vi "Graph Value to IMAQ Image.vi"(7 "Gray?":bool, 8 "error in":errorcluster, 11 "Intensity Graph Refnum":refnum<vi>) -> (0 "error out":errorcluster, 3 "IMAQ Image":T1)   [LabVIEW 2025, in "Base Graph.lvclass"]
uses:
  Base Graph.lvclass
  <vilib>/vision/Image Controls.llb/IMAQ Image.ctl
  Open-Xml-LabVIEW/Common-Labview-helpers/Source/Common Helpers.lvlib
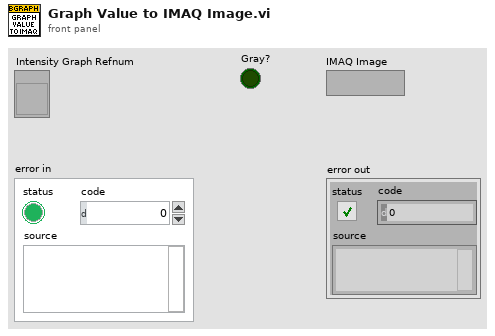
[diagram p1: front panel]
types:
  T1 = typedef "IMAQ Image.ctl" = refnum<image>
  T2 = typedef "Image Type" = u32
  T3 = typedef "imagedata.ctl" = cluster{"image type":i32, "image depth":i32, "image":u8[], "mask":u8[], "colors":u32[], "Rectangle":cluster{"left":i16, "top":i16, "right":i16, "bottom":i16}}
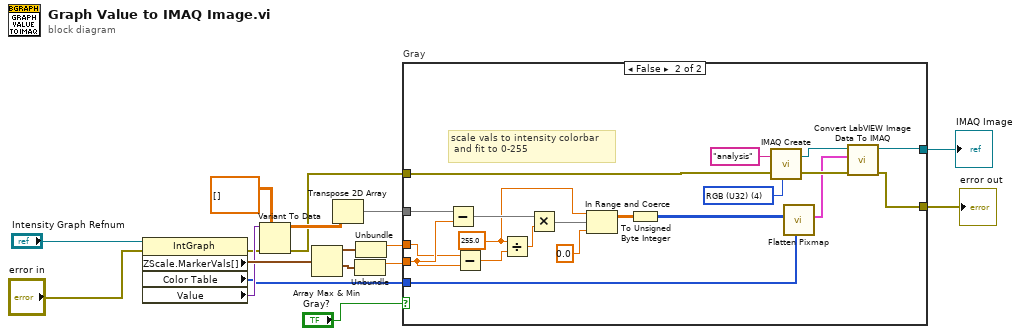
[diagram p0: block diagram]
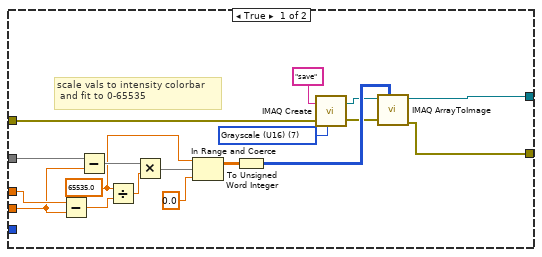
[diagram p2: hidden frame]
diagram:
  n1 = property class="IntGraph"(reference="Intensity Graph Refnum", error in="error in") -> (error out=w11:errorcluster, "ZScale.MarkerVals[]"=w14:cluster{dbl, u32}[], "Color Table"=w2:u32[], "Value"=w12:variant)  [unwired: 1 out]
  n2 = Variant To Data(error in=w11, type=dbl[][] [], Variant=w12) -> (data=w10:dbl[][], error out=w5:errorcluster)
  n3 = Array Max & Min(array=w14) -> (max value=w15:cluster{dbl, u32}, min value=w16:cluster{dbl, u32})  [unwired: 2 out]
  n4 = Transpose 2D Array(2D array=w10) -> (transposed array=w6:dbl[][])
  n5 = Unbundle(w16) -> (w8:dbl)  [unwired: 1 out]
  n6 = Unbundle(w15) -> (w7:dbl)  [unwired: 1 out]
  n7 = case "Gray" shown="False" "Gray?" {
    tunnel: w6 -> [w27 w47]
    tunnel: w5 -> [w26 w46]
    tunnel: [w25 w36] -> w3
    tunnel: [w24 w37] -> w4
    tunnel: w8 -> [w22 w45]
    tunnel: w7 -> [w23 w44]
    tunnel: w2 -> [_ w41]
    frame True {
      w18 = T2 7 items=["Grayscale (U8)", "Grayscale (I16)", "Grayscale (SGL)", "Complex (CSG)", "RGB (U32)", "HSL (U32)", "RGB (U64)", "Grayscale (U16)"] ("Image Type")
      w31 = 65535.0
      # "scale vals to intensity colorbar\n and fit to 0-65535"
      n8 = Subtract(x=w23, y=w22) -> (x-y=w34:dbl)
      n9 = Subtract(x=w27, y=w22) -> (x-y=w35:dbl[][])
      n10 = Divide(x=w31, y=w34) -> (x/y=w33:dbl)
      n11 = Multiply(x=w35, y=w33) -> (x*y=w30:dbl[][])
      n12 = In Range and Coerce(upper limit=w31, x=w30, lower limit=0.0) -> (coerced(x)=w29:dbl[][])  [unwired: 1 out]
      n13 = To Unsigned Word Integer(number=w29) -> (unsigned 16bit integer=w28:u16[][])
      n14 = call "IMAQ Create"("Image Name"="save", "Image Type"=w18, "error in (no error)"=w26) -> ("New Image"=w20:T1, "error out"=w21:errorcluster)  [unwired: 2 in]
      n15 = call "IMAQ ArrayToImage"("Image Pixels (U16)"=w28, "error in (no error)"=w21, "Image"=w20) -> ("error out"=w25:errorcluster, "Image Out"=w24:T1)  [unwired: 7 in]
    }
    frame False {
      w42 = T2 4 items=["Grayscale (U8)", "Grayscale (I16)", "Grayscale (SGL)", "Complex (CSG)", "RGB (U32)", "HSL (U32)", "RGB (U64)", "Grayscale (U16)"] ("Image Type")
      w51 = 255.0
      # "scale vals to intensity colorbar\n and fit to 0-255"
      n16 = Subtract(x=w47, y=w45) -> (x-y=w55:dbl[][])
      n17 = Subtract(x=w44, y=w45) -> (x-y=w54:dbl)
      n18 = Divide(x=w51, y=w54) -> (x/y=w53:dbl)
      n19 = Multiply(x=w55, y=w53) -> (x*y=w50:dbl[][])
      n20 = In Range and Coerce(upper limit=w51, x=w50, lower limit=0.0) -> (coerced(x)=w49:dbl[][])  [unwired: 1 out]
      n21 = To Unsigned Byte Integer(number=w49) -> (unsigned 8bit integer=w48:u8[][])
      n22 = call "IMAQ Create"("Image Name"="analysis", "Image Type"=w42, "error in (no error)"=w46) -> ("New Image"=w39:T1, "error out"=w40:errorcluster)  [unwired: 2 in]
      n23 = call <vilib>:"Flatten Pixmap.vi"("colors"=w41, "8-bit pixmap"=w48) -> ("image data"=w38:T3)  [unwired: 9 in]
      n24 = call "Convert LabVIEW Image Data To IMAQ.vi"("error in"=w40, "Image Data"=w38, "Image In"=w39) -> ("error out"=w36:errorcluster, "Image Out"=w37:T1)  [unwired: 7 in]
    }
  }
  "error out" <- w3
  "IMAQ Image" <- w4
